vi "Get Resource from Connection UI Element.vi"(10 "Connection Element":string, 11 "Alias Mappings by Module":T1(array[cluster])) -> (2 "Endpoint":string, 3 "Resource":string)   [LabVIEW 2017, in "Routing and Faulting System Explorer.lvlib"]
uses:
  Routing and Faulting System Explorer.lvlib
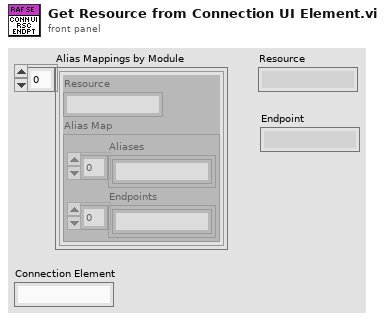
[diagram p1: front panel]
types:
  T1 = cluster{"Resource":string, "Alias Map":cluster{"Aliases":string[], "Endpoints":string[]}}[]
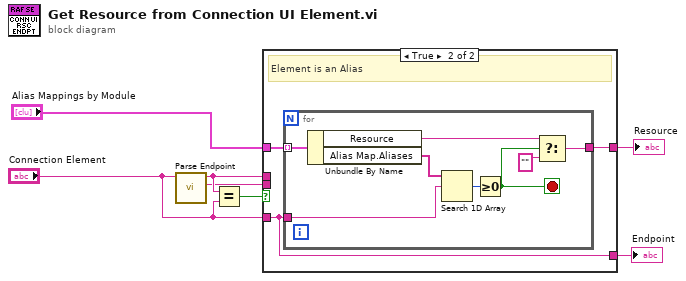
[diagram p0: block diagram]
diagram:
  n1 = call "Parse Endpoint.vi"("Resource/Endpoint"="Connection Element") -> ("Endpoint"=w2:string, "Resource"=w4:string)  [unwired: 9 in]
  n2 = Equal?(x=w4, y="Connection Element") -> (x = y?=w3:bool)
  n3 = case shown="True" w3 {
    tunnel: "Alias Mappings by Module" -> [_ w12]
    tunnel: w4 -> [w9 _]
    tunnel: [w9 w11] -> w7
    tunnel: "Connection Element" -> [_ w10]
    tunnel: [w8 w10] -> w1
    tunnel: w2 -> [w8 _]
    frame False {
      # "Element is in Resource/Endpoint format"
    }
    frame True {
      # "Element is an Alias"
      n4 = for {
        tunnel: w12 -> [w20] mode=indexing
        tunnel: w10 -> [w17]
        tunnel: [w13] -> w11
        stop <- w16 stop-if-true
        n5 = Unbundle By Name(w20) -> ("Resource"=w14:string, "Alias Map.Aliases"=w19:string[])
        n6 = Search 1D Array(1D array=w19, element=w17) -> (index of element=w18:i32)  [unwired: 1 in]
        n7 = Greater Or Equal To 0?(x=w18) -> (x >= 0?=w16:bool)
        n8 = Select(t=w14, s=w16, f="") -> (s? t:f=w13:string)
      }
    }
  }
  "Resource" <- w7
  "Endpoint" <- w1
